vi "WCA_CAN_close.vi"(2 "ObjHandle in":u32, 11 "error in (no error)":errorcluster) -> (15 "error out":errorcluster)   [LabVIEW 2017]
uses:
  WCA_Global.vi
panel:
  out "Slave Node in":cluster{"Address":i16, "Serial Number":i8[]} {"Serial Number" format="%.0x"; "Address" format="%.0x"}
  # "Node Address"
  # "Serial Number"
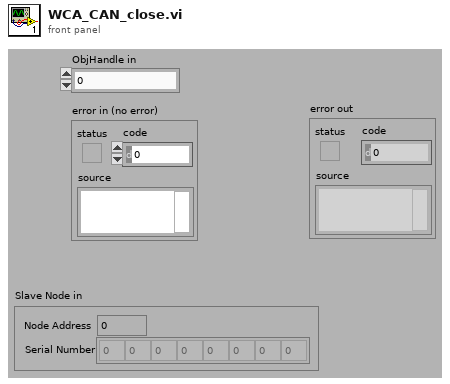
[diagram p1: front panel]
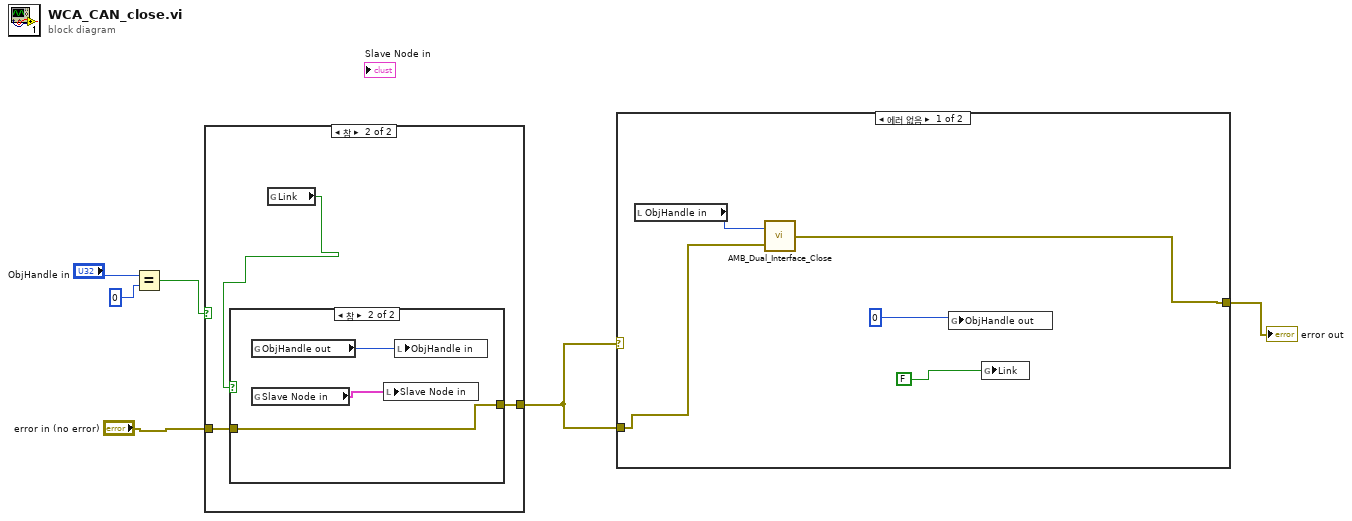
[diagram p0: block diagram]
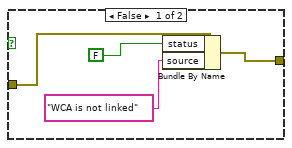
[diagram p4: hidden frame]
diagram:
  n1 = Equal?(x="ObjHandle in", y=0) -> (x = y?=w4:bool)
  n2 = case shown="참" w4 {
    tunnel: "error in (no error)" -> [w7 w10]
    tunnel: [w7 w9] -> w2
    frame False {
    }
    frame True {
      n3 = global read "WCA_Global.vi" "Link"() -> (w8:bool)
      n4 = case shown="참" w8 {
        tunnel: w10 -> [w14 w15]
        tunnel: [w11 w15] -> w9
        frame False {
          n5 = Bundle By Name(cluster=w14, "status"=FALSE, "source"="WCA is not linked") -> (w11:errorcluster)
        }
        frame True {
          n6 = global read "WCA_Global.vi" "ObjHandle out"() -> (w17:u32)
          n7 = global read "WCA_Global.vi" "Slave Node in"() -> (w16:cluster{"Address":i16, "Serial Number":i8[]})
          n8 = local write "Slave Node in"(w16) -> ()
          n9 = local write "ObjHandle in"(w17) -> ()
        }
      }
    }
  }
  n10 = case shown="에러 없음" w2 {
    tunnel: w2 -> [w21 w23]
    tunnel: [w20 w23] -> w1
    frame No Error {
      n11 = local read "ObjHandle in"() -> (w22:u32)
      n12 = call "AMB_Dual_Interface_Close.vi"("Error In"=w21, "Object\nHandle"=w22) -> ("Error Out"=w20:errorcluster)
      n13 = global write "WCA_Global.vi" "ObjHandle out"(0) -> ()
      n14 = global write "WCA_Global.vi" "Link"(FALSE) -> ()
    }
    frame Error {
    }
  }
  "error out" <- w1
